vi "Less Than Float SCTL 40 MHz Latency 0 Pipeline 0.vi"(1 "y":sgl, 2 "x":sgl) -> (0 "x < y?":bool)   [LabVIEW 2015]
uses:
  <vilib>/rvi/IPIntegrationNode/IPINode_Typedef/niFpgaIPINodeSupportedFamilies.ctl
  <vilib>/rvi/IPIntegrationNode/IPINode_Utilities/niFpgaIPINodeSimCore.vi
  <vilib>/rvi/XilinxIP/XIPIN_XNode/niFpgaXIPIN.xnode
  Compare SCTL/Compare_SCTL_C3ADE5BE76064AA39E7EE6565DE88692.dll
  <vilib>/rvi/IPIntegrationNode/IPINode_Xnode/niFpgaIPINode.xnode
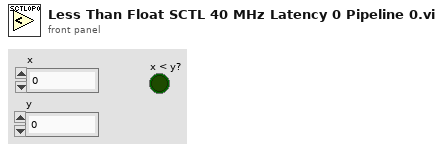
[diagram p1: front panel]
types:
  T1 = typedef "niFpgaIPINodeSupportedFamilies.ctl" = cluster{"unlimited?":bool, "supported targets":string[]}
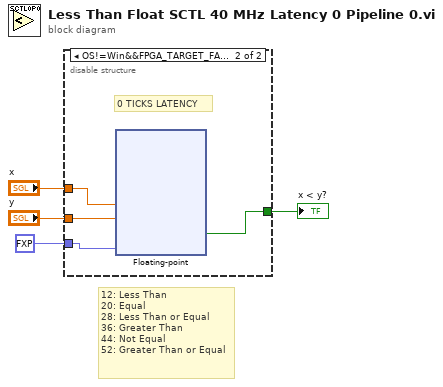
[diagram p0: block diagram]
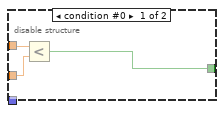
[diagram p2: hidden frame]
diagram:
  # "12: Less Than\n20: Equal\n28: Less Than or Equal\n36: Greater Than\n44: Not Equal\n52: Greater Than or Equal"
  n1 = disable-structure shown="OS!=Win&&FPGA_TARGET_FAMILY==SPARTAN6" {
    disable-tunnel: "x" -> [w6 w11]
    disable-tunnel: "y" -> [w5 w10]
    disable-tunnel: [w7 w9] -> w1
    disable-tunnel: fxp<+,8,8> 12.0 ("s_axis_operation_tdata") -> [_ w8]
    frame condition #0 {
      n2 = Less?(x=w6, y=w5) -> (x < y?=w7:bool)
    }
    frame condition #1 (active) {
      # "0 TICKS LATENCY"
      n3 = xnode ("Floating-point")("a"=w11, "b"=w10, "operation"=w8) -> ("result"=w9:bool)
    }
  }
  "x < y?" <- w1
